vi "Create All Message Queues.vi"(8 "error in (no error)":errorcluster) -> (0 "error out":errorcluster, 3 "Message Queues out":T1)   [LabVIEW 2024, in "Message Queue.lvlib"]
doc: "This VI creates and initializes all the message queues for your application. If your application requires more than one message queue, right-click the \"Message Queues\" constant above and select Open Type Def. Add the new Message Queue(s) to the type definition, then initialize them in this VI."
uses:
  Message Queue.lvlib
  All Message Queues.ctl
  Message Cluster.ctl
  Enqueue Message (Single).vi
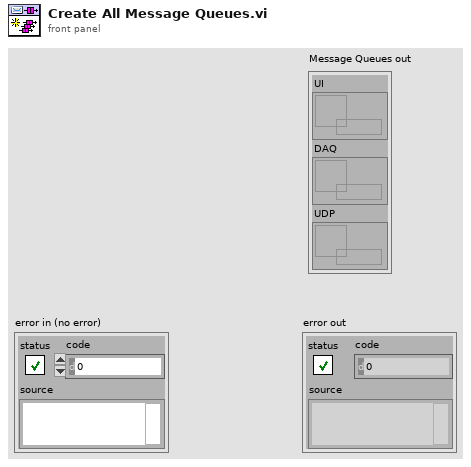
[diagram p1: front panel]
types:
  T1 = typedef "Message Queue.lvlib/All Message Queues.ctl" = cluster{"UI":refnum<queue>, "DAQ":refnum<queue>, "UDP":refnum<queue>}
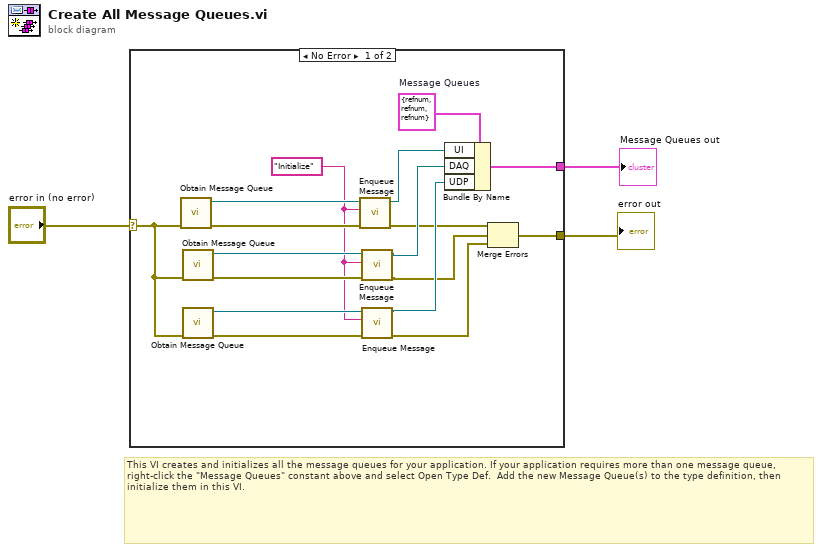
[diagram p0: block diagram]
diagram:
  # "This VI creates and initializes all the message queues for your application. If your application requires more than one message queue, right-click the \"Message Queues\" constant above and select Open Type Def.  Add the new Message Queue(s) to the type definition, then initialize them in this VI."
  n1 = case shown="No Error" "error in (no error)" {
    selector: "error in (no error)" -> [w13 w21]
    tunnel: [w4 w21] -> w3
    tunnel: [w19 _] -> w2
    frame No Error {
      w10 = "Initialize" ("Message")
      w20 = T1 {"UI"=refnum, "DAQ"=refnum, "UDP"=refnum}  # Message Queues
      n2 = call "Obtain Message Queue.vi"("error in (no error)"=w13) -> ("error out"=w18:errorcluster, "Message Queue"=w17:refnum<queue>)  [unwired: 9 in]
      n3 = call "Obtain Message Queue.vi"("error in (no error)"=w13) -> ("error out"=w15:errorcluster, "Message Queue"=w12:refnum<queue>)  [unwired: 9 in]
      n4 = call "Obtain Message Queue.vi"("error in (no error)"=w13) -> ("error out"=w14:errorcluster, "Message Queue"=w11:refnum<queue>)  [unwired: 9 in]
      n5 = call-poly "Enqueue Message.vi"("error in (no error)"=w18, "Message"=w10, "Message Queue"=w17) -> ("error out"=w7:errorcluster, "dup Message Queue"=w16:refnum<queue>)  [unwired: 7 in]
      n6 = call-poly "Enqueue Message.vi"("error in (no error)"=w15, "Message"=w10, "Message Queue"=w12) -> ("error out"=w6:errorcluster, "dup Message Queue"=w9:refnum<queue>)  [unwired: 7 in]
      n7 = call-poly "Enqueue Message.vi"("error in (no error)"=w14, "Message"=w10, "Message Queue"=w11) -> ("error out"=w5:errorcluster, "dup Message Queue"=w8:refnum<queue>)  [unwired: 7 in]
      n8 = Bundle By Name(cluster=w20, "UI"=w16, "DAQ"=w9, "UDP"=w8) -> (w19:T1)
      n9 = Merge Errors(w7, w6, w5) -> (w4:errorcluster)
    }
    frame Error {
    }
  }
  "Message Queues out" <- w2
  "error out" <- w3
